vi "DeleteWfrms.vi"(8 "error in (no error)":errorcluster, 10 "NumRecords":i32, 11 "FunctionBase in":refnum<class "FunctionBase.lvclass">) -> (0 "error out":errorcluster, 2 "DeletedWaveforms":waveform(dbl)[](array[waveform]), 3 "FunctionBase out":refnum<class "FunctionBase.lvclass">)   [LabVIEW 2014, in "Functions.lvlib" / "FunctionBase.lvclass"]
uses:
  FunctionBase.lvclass
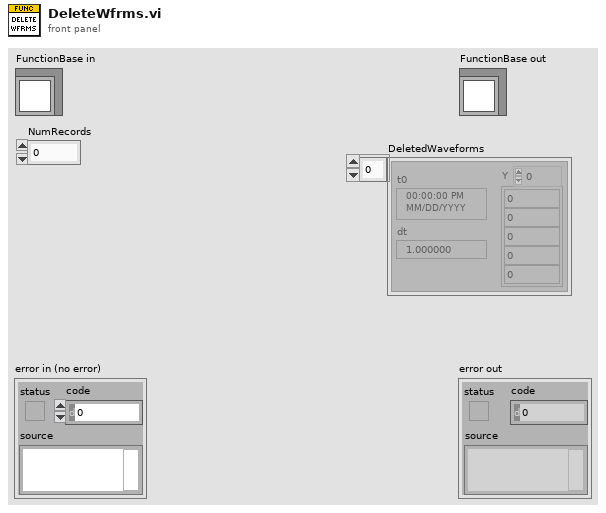
[diagram p1: front panel]
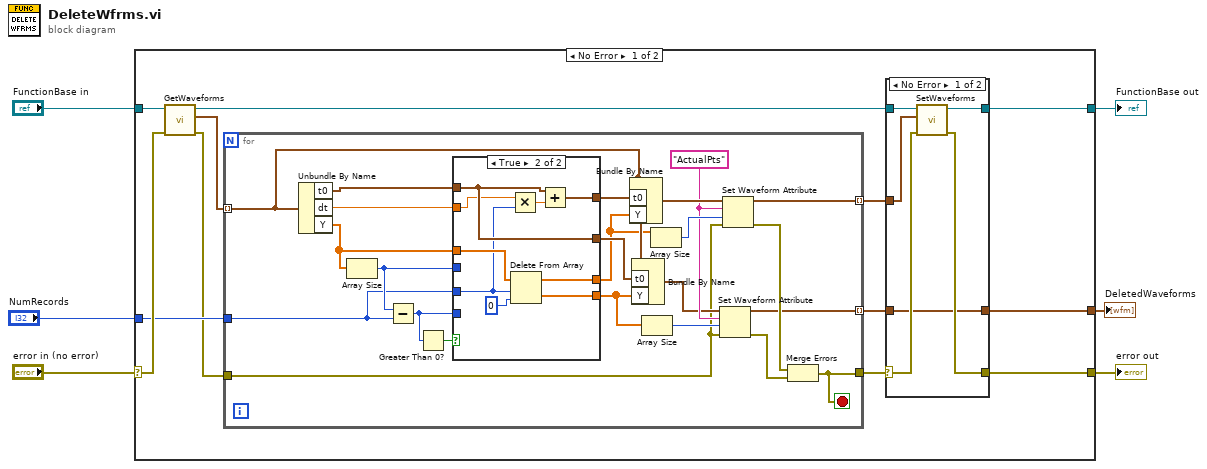
[diagram p0: block diagram]
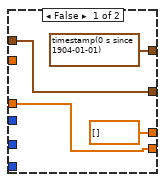
[diagram p3: hidden frame]
diagram:
  n1 = case shown="No Error" "error in (no error)" {
    selector: "error in (no error)" -> [w17 w64]
    tunnel: [w9 w64] -> w5
    tunnel: [w10 w63] -> w3
    tunnel: "FunctionBase in" -> [w18 w63]
    tunnel: "NumRecords" -> [w15 _]
    tunnel: [w7 _] -> w1
    frame No Error {
      n2 = call-dynamic "GetWaveforms.vi"("error in (no error)"=w17, "FunctionBase in"=w18) -> ("error out"=w14:errorcluster, "Waveforms"=w16:waveform(dbl)[], "FunctionBase out"=w12:refnum<class "FunctionBase.lvclass">)  [unwired: 7 in]
      n3 = for {
        tunnel: w16 -> [w40] mode=indexing
        tunnel: w15 -> [w46]
        tunnel: w14 -> [w32]
        tunnel: [w29] -> w13
        tunnel: [w28] -> w11 mode=indexing
        tunnel: [w27] -> w8 mode=indexing
        stop <- w29 stop-if-true
        w36 = "ActualPts"
        n4 = Unbundle By Name(w40) -> ("t0"=w43:timestamp, "dt"=w44:dbl, "Y"=w45:dbl[])
        n5 = Array Size(array=w45) -> (size(s)=w47:i32)
        n6 = Subtract(x=w47, y=w46) -> (x-y=w48:i32)
        n7 = Greater Than 0?(x=w48) -> (x > 0?=w49:bool)
        n8 = case shown="True" w49 {
          tunnel: w48 -> [_ _]
          tunnel: w47 -> [_ _]
          tunnel: w46 -> [_ w54]
          tunnel: w45 -> [w50 w61]
          tunnel: [dbl[] [] ("Y") w60] -> w39
          tunnel: [w50 w59] -> w35
          tunnel: w44 -> [_ w55]
          tunnel: w43 -> [w52 w56]
          tunnel: [timestamp(0 s since 1904-01-01) w57] -> w42
          tunnel: [w52 w56] -> w41
          frame False {
          }
          frame True {
            n9 = Multiply(x=w55, y=w54) -> (x*y=w58:dbl)
            n10 = Delete From Array(array=w61, length=w54, index=0) -> (deleted portion=w59:dbl[], array with subset deleted=w60:dbl[])
            n11 = Add(x=w56, y=w58) -> (x+y=w57:timestamp)
          }
        }
        n12 = Bundle By Name(cluster=w40, "t0"=w42, "Y"=w39) -> (w37:waveform(dbl))
        n13 = Bundle By Name(cluster=w40, "t0"=w41, "Y"=w35) -> (w33:waveform(dbl))
        n14 = Array Size(array=w35) -> (size(s)=w34:i32)
        n15 = Array Size(array=w39) -> (size(s)=w38:i32)
        n16 = Set Waveform Attribute(4:w32, 5:w34, 6:w36, 7:w33) -> (0:w31:errorcluster, 3:w27:waveform(dbl))  [unwired: 1 out]
        n17 = Set Waveform Attribute(4:w32, 5:w38, 6:w36, 7:w37) -> (0:w30:errorcluster, 3:w28:waveform(dbl))  [unwired: 1 out]
        n18 = Merge Errors(w30, w31) -> (w29:errorcluster)
      }
      n19 = case shown="No Error" w13 {
        selector: w13 -> [w22 w26]
        tunnel: w12 -> [w24 w25]
        tunnel: w11 -> [w23 _]
        tunnel: [w21 w25] -> w10
        tunnel: [w20 w26] -> w9
        tunnel: w8 -> [w19 _]
        tunnel: [w19 _] -> w7
        frame No Error {
          n20 = call-dynamic "SetWaveforms.vi"("error in (no error)"=w22, "Waveforms"=w23, "FunctionBase in"=w24) -> ("error out"=w20:errorcluster, "FunctionBase out"=w21:refnum<class "FunctionBase.lvclass">)  [unwired: 7 in]
        }
        frame Error {
        }
      }
    }
    frame Error {
    }
  }
  "error out" <- w5
  "FunctionBase out" <- w3
  "DeletedWaveforms" <- w1
